vi "RT_interface.vi"() -> ()   [LabVIEW 2019]
uses:
  <vilib>/Platform/TimedLoop/XDataNode/timing_clust.ctl
  <vilib>/Platform/TimedLoop/XDataNode/nitl_modes.ctl
  <vilib>/Platform/TimedLoop/XDataNode/wakeup.ctl
  <vilib>/FPGAPlugInAG/myRIO-1900/niLvFpga_Open_myRIO-1900.vi
  <vilib>/rvi/interface/common/dynamic/niFpgaDynamicAddResources.vi
  <vilib>/Utility/error.llb/Error Cluster From Error Code.vi
  <vilib>/rvi/errors/niLvFpgaAdjustHostInterfaceError.vi
  <vilib>/FPGAPlugInAG/Dynamic/niLvFpga_Close_Dynamic.vi
  <vilib>/platform/TimedLoop/XDataNode/XDataNode.xnode
  <vilib>/rvi/interface/nirviOpenFPGA/nirviOpenFPGA.xnode
  catheter20210803_FPGATarget_PPGAdriver_RvkUSVpzf1Y.lvbitx
  <vilib>/rvi/interface/nirviReadWriteControl/nirviReadWriteControl.xnode
  <vilib>/rvi/interface/nirviCloseFPGA/nirviCloseFPGA.xnode
  <vilib>/Platform/TimedLoop/XDataNode/XDNodeRunTimeDep.lvlib
  <vilib>/rvi/interface/Simulation/niFpgaSimulationCallBeginRW.vi
  NiFpgaLv.dll
panel:
  out "ConnectorC/AO0":i16
  out "ConnectorC/AO1":i16
  out "Duty Ratio":dbl
  out "stepper position":i32(graph)=-58
  out "PWM coil":dbl(graph)
  in  "Steering gain":dbl=1.0
  in  "Pushing Gain":dbl=-0.5
  in  "Enable stepper?":bool=TRUE
  out "Encoder 2 reading":i16(graph)=-924
  out "Encoder 1 reading":i16(graph)=-115
  out "Encoder1  Position":i16=-115
  in  "stop":bool
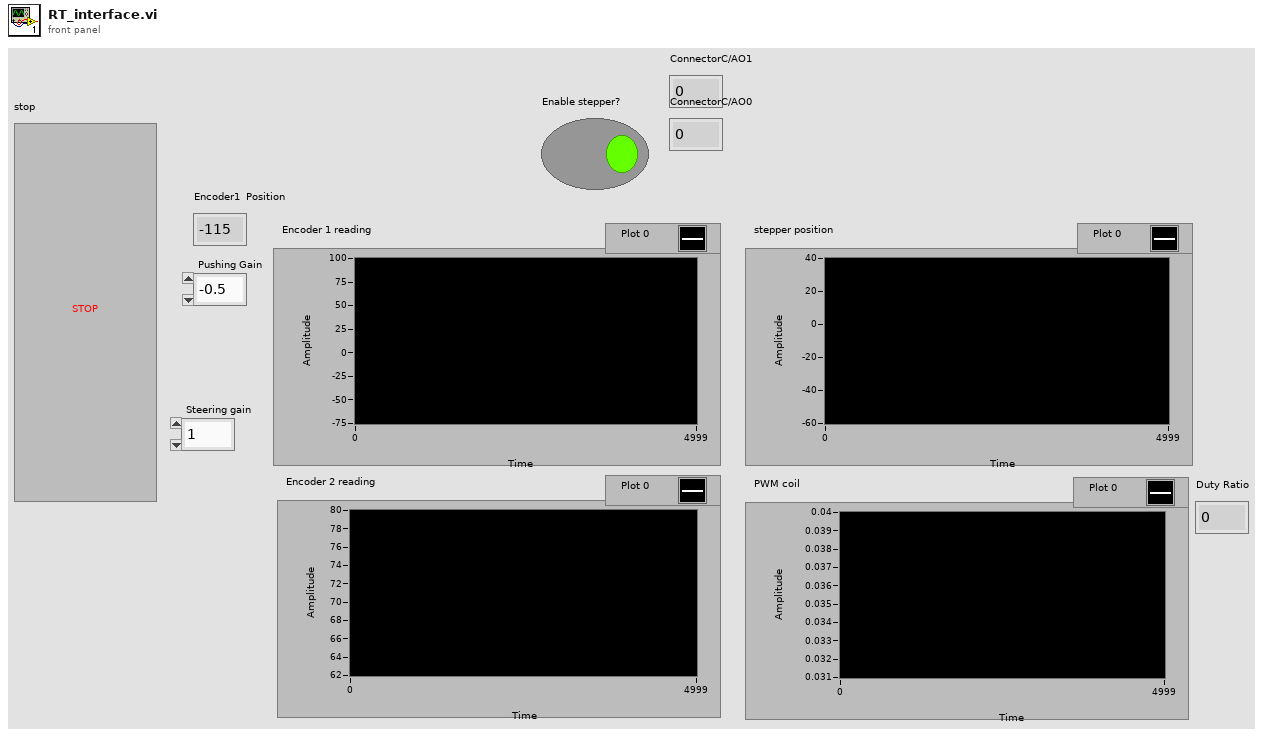
[diagram p1: front panel]
types:
  T1 = typedef "XDNodeRunTimeDep.lvlib/timing_clust.ctl" = cluster{"Expected End [f-1]":u64, "Actual End [f-1]":u64, "Finished Late? [f-1]":bool, "Expected End [i-1]":u64, "Actual End [i-1]":u64, "Finished Late? [i-1]":bool, "Expected Start [i]":u64, "Actual Start [i]":u64, "Expected Start [f]":u64, "Actual Start [f]":u64, "Source Name":string, "Structure Name":string, "Period":i64, "Deadline":i64, "Offset":i64, "Start":i64, "Priority":i32, "Timeout":i32, "Mode":T2, "Wakeup Reason":T3, "Error":errorcluster, "Source Type":string, "Secondary Source Type":string, "Global End Time":u64, "Global Start Time":u64, "Frame Duration":u64, "Iteration Duration":u64, "Assigned CPU":i32, "I/O Scan Engine Mode":u32}
  T2 = typedef "XDNodeRunTimeDep.lvlib/nitl_modes.ctl" = enum32{"No Change", "Process missed periods, maintain original phase", "Discard missed periods, maintain original phase", "Process missed periods, ignore original phase", "Discard missed periods, ignore original phase"}
  T3 = typedef "XDNodeRunTimeDep.lvlib/wakeup.ctl" = enum32{"Normal", "Aborted", "Asynchronous wakeup", "Timing source error", "Timed loop error", "Timeout"}
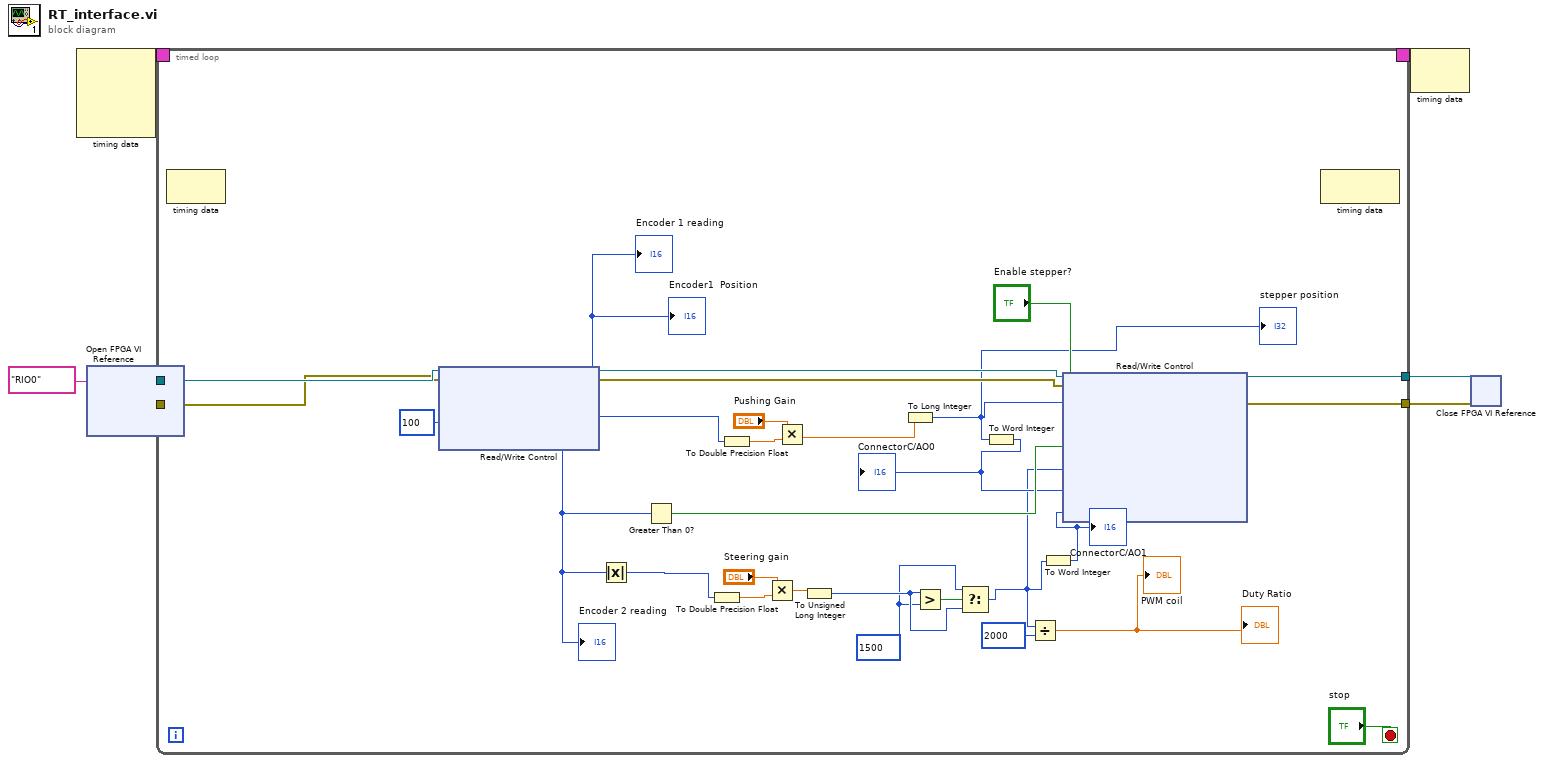
[diagram p0: block diagram]
diagram:
  n1 = node-c288() -> (w7:T1)  [unwired: 4 in]
  n2 = xnode "Open FPGA VI Reference"("resource name"=tag "RIO0") -> ("FPGA VI Reference Out"=w5:refnum<k20>, "error out"=w4:errorcluster)  [unwired: 1 in]
  n3 = timed-loop {
    timing: w7 -> [_]
    timing-out: [_] -> w6
    tunnel: w5 -> [w15]
    tunnel: w4 -> [w14]
    tunnel: [w33] -> w3
    tunnel: [w32] -> w2
    stop <- "stop" stop-if-true
    w17 = u32 1500 ("y")
    n4 = node-c288() -> ()  [unwired: 1 in, 1 out]
    n5 = xnode "Read/Write Control"("FPGA VI Reference In"=w15, "error in"=w14, "Velocity  Limit"=100) -> ("FPGA VI Reference Out"=w34:refnum<k20>, "error out"=w13:errorcluster, "Encoder Position"=w30:i16, "Encoder Position 2"=w21:i16)
    "Encoder1  Position" <- w30
    "Encoder 1 reading" <- w30
    "Encoder 2 reading" <- w21
    n6 = Absolute Value(x=w21) -> (abs(x)=w22:i16)
    n7 = Greater Than 0?(x=w21) -> (x > 0?=w26:bool)
    n8 = To Double Precision Float(number=w22) -> (double precision float=w24:dbl)
    n9 = To Double Precision Float(number=w30) -> (double precision float=w29:dbl)
    n10 = Multiply(x="Steering gain", y=w24) -> (x*y=w20:dbl)
    n11 = Multiply(x="Pushing Gain", y=w29) -> (x*y=w27:dbl)
    n12 = To Unsigned Long Integer(number=w20) -> (unsigned 32bit integer=w18:u32)
    n13 = To Long Integer(number=w27) -> (32bit integer=w12:i32)
    "stepper position" <- w12
    n14 = Greater?(x=w18, y=w17) -> (0:w19:bool)
    n15 = Select(t=w17, s=w19, f=w18) -> (s? t:f=w10:u32)
    n16 = To Word Integer(number=w12) -> (16bit integer=w11:i16)
    "ConnectorC/AO0" <- w11
    n17 = Divide(x=w10, y=u32 2000) -> (x/y=→"PWM coil" →"Duty Ratio":dbl)
    n18 = To Word Integer(number=w10) -> (16bit integer=w8:i16)
    "ConnectorC/AO1" <- w8
    n19 = xnode "Read/Write Control"("FPGA VI Reference In"=w34, "error in"=w13, "Position Ref."=w12, "enable?"="Enable stepper?", "Coil Current Direction"=w26, "Num_cycle_on"=w10, "ConnectorC/AO0"=w11, "ConnectorC/AO1"=w8) -> ("FPGA VI Reference Out"=w33:refnum<k20>, "error out"=w32:errorcluster)
    n20 = node-c288() -> ()  [unwired: 1 in, 1 out]
  }
  n21 = node-c288(w6) -> ()  [unwired: 1 out]
  n22 = xnode "Close FPGA VI Reference"("FPGA VI Reference In"=w3, "error in"=w2) -> ()  [unwired: 1 out]
